vi "Out_S2F24.vi"(8 "error in (no error)":errorcluster, 10 "S2F24":T1, 11 "S2 Message Class in":refnum<class "S2 Message Class.lvclass">) -> (0 "error out":errorcluster, 3 "S2 Message Class out":refnum<class "S2 Message Class.lvclass">)   [LabVIEW 2020, in "SECS Communication.lvlib" / "S2 Message Class.lvclass"]
uses:
  S2 Message Class.lvclass
  D:/Dropbox/SECS/SECS_GEM v1.0.6/Com/SECS Communication/SECS-II Class/SECS-II Class.lvclass
  S2F24.ctl
  SECS-II Class/Data Message_Binary.vi
  SECS-II Class/SECS-II Class.lvclass
  D:/Dropbox/SECS/SECS_GEM v1.0.6/Com/SECS Communication/S2 Message Class/S2 Message Class.lvclass
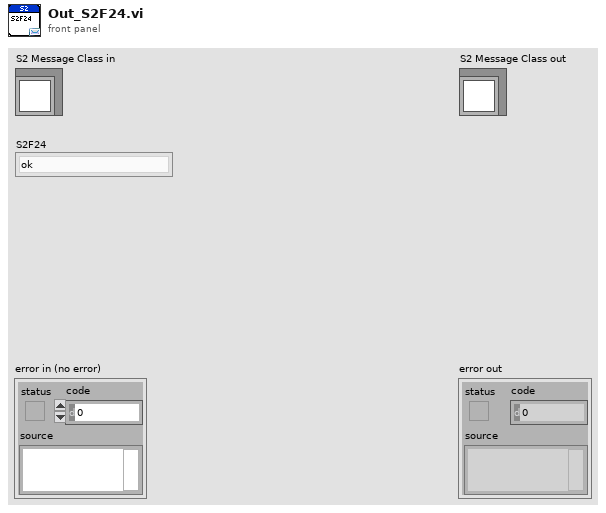
[diagram p1: front panel]
types:
  T1 = typedef "SECS Communication.lvlib/S2 Message Class.lvclass/S2F24.ctl" = enum16{"ok", "too many SVIDs", "no more traces allowed", "invalid period", "unknown SVID", "bad REPGSZ"}
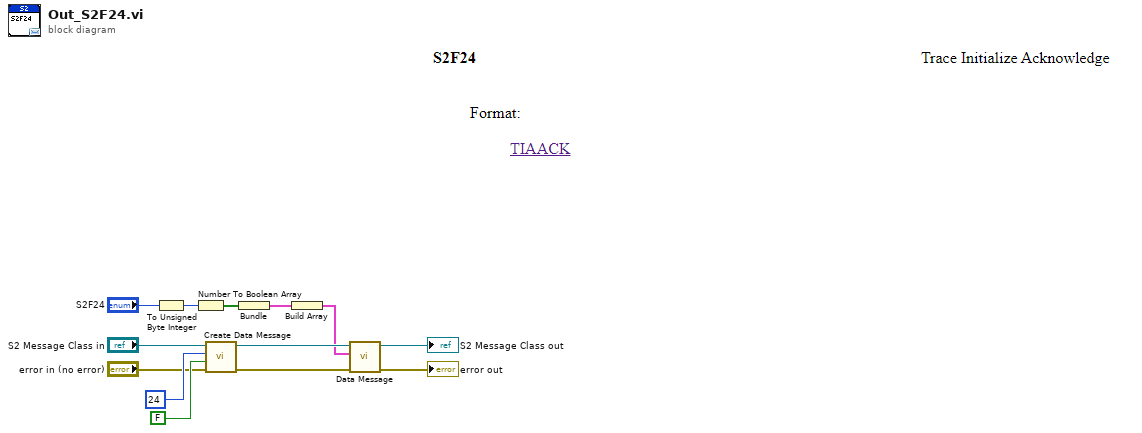
[diagram p0: block diagram]
diagram:
  n1 = To Unsigned Byte Integer(number="S2F24") -> (unsigned 8bit integer=w4:u8)
  n2 = Number To Boolean Array(number=w4) -> (Boolean array=w3:bool[])
  n3 = call "Create Data Message.vi"("error in (no error)"="error in (no error)", "W-Bit"=FALSE, "Function"=u8 24, "SECS-II Class in"="S2 Message Class in") -> ("error out"=w10:errorcluster, "SECS-II Class out"=w11:refnum<class "S2 Message Class.lvclass">)  [unwired: 6 in]
  n4 = Bundle("Boolean array"=w3) -> (w2:cluster{"Boolean array":bool[]})  [unwired: 1 in]
  n5 = Build Array(w2) -> (w1:cluster{"Boolean array":bool[]}[])
  n6 = call-poly "Data Message.vi"("error in"=w10, "Data Cluster"=w1, "SECS-II Class in"=w11) -> ("error out"=→"error out":errorcluster, "SECS-II Class out"=→"S2 Message Class out":refnum<class "S2 Message Class.lvclass">)  [unwired: 7 in]
